vi "获取组列表.vi"(8 "错误输入（无错误）":errorcluster, 11 "引用句柄输入":refnum<k34>) -> (0 "错误输出":errorcluster, 2 "组列表":string[](array[string]), 3 "引用句柄输出":refnum<k34>)   [LabVIEW 2021]
uses:
  a17fec19-d12b-4b71-ae4f-b091a59b9431.vi
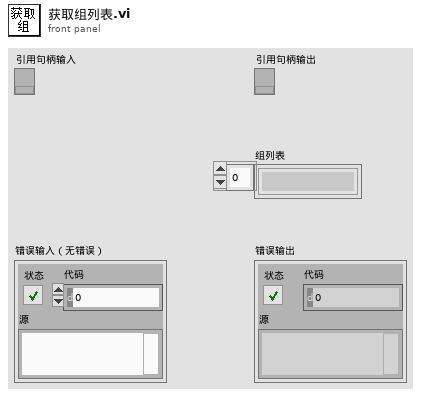
[diagram p1: front panel]
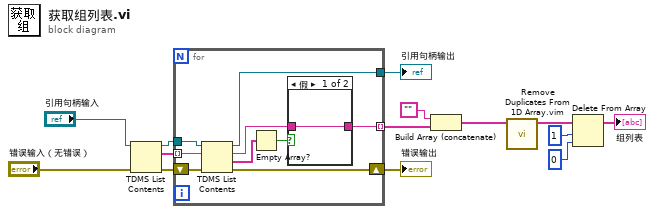
[diagram p0: block diagram]
diagram:
  n1 = TDMS List Contents(4:"错误输入（无错误）", 7:"引用句柄输入") -> (0:w5:errorcluster, 2:w4:string[], 3:w3:refnum<k34>)  [unwired: 1 in, 1 out]
  n2 = for {
    tunnel: w3 -> [w23]
    tunnel: w4 -> [w22] mode=indexing
    tunnel: [w18] -> w13
    tunnel: [w16] -> w7 mode=indexing
    shift-right: [w15] -> w14
    shift-left: w5 -> [w21]
    n3 = TDMS List Contents(4:w21, 6:w22, 7:w23) -> (0:w15:errorcluster, 1:w20:string[], 2:w17:string, 3:w18:refnum<k34>)
    n4 = Empty Array?(array=w20) -> (empty?=w19:bool)
    n5 = case shown="假" w19 {
      tunnel: w17 -> [w24 _]
      tunnel: [w24 _] -> w16
      frame False {
      }
      frame True {
      }
    }
  }
  "错误输出" <- w14
  "引用句柄输出" <- w13
  n6 = Build Array (concatenate)("", w7) -> (w8:string[])
  n7 = call "Remove Duplicates From 1D Array.vim"("array"=w8) -> ("array with duplicates removed"=w9:string[])  [unwired: 10 in]
  n8 = Delete From Array(array=w9, length=1 ("长度"), index=0 ("索引")) -> (array with subset deleted=→"组列表":string[])  [unwired: 1 out]
